vi "Facade.vi"(0 "Data In":T4, 2 "Display State In":T2, 3 "Container State":T3) -> (6 "Data Out":T4, 7 "Display State Out":T2, 8 "Action":T1)   [LabVIEW 2011, in "BlinkingButton.xctl"]
uses:
  <vilib>/_probes/SAPHIR/ViBox - Probes/BlinkingButton/BlinkingButton.xctl
  <vilib>/_probes/SAPHIR/ViBox - Probes/BlinkingButton/Data.ctl
  <vilib>/_xctls/Container State.ctl
  <vilib>/_probes/SAPHIR/ViBox - Probes/BlinkingButton/State.ctl
  <vilib>/_xctls/Action.ctl
  <vilib>/_xctls/XControlSupport.lvlib
panel:
  in  "FreezeDisplay":bool
  out "Blinker":bool
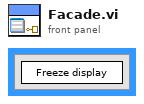
[diagram p1: front panel]
types:
  T1 = typedef "XControlSupport.lvlib/Action.ctl" = cluster{"Data Changed?":bool, "State Changed?":bool, "Action Name":string}
  T2 = typedef "BlinkingButton.xctl/State.ctl" = cluster{"Numeric":dbl}
  T3 = typedef "XControlSupport.lvlib/Container State.ctl" = cluster{"Indicator?":bool, "Run Mode?":bool, " Refnum":refnum<vi>}
  T4 = typedef "BlinkingButton.xctl/Data.ctl" = bool
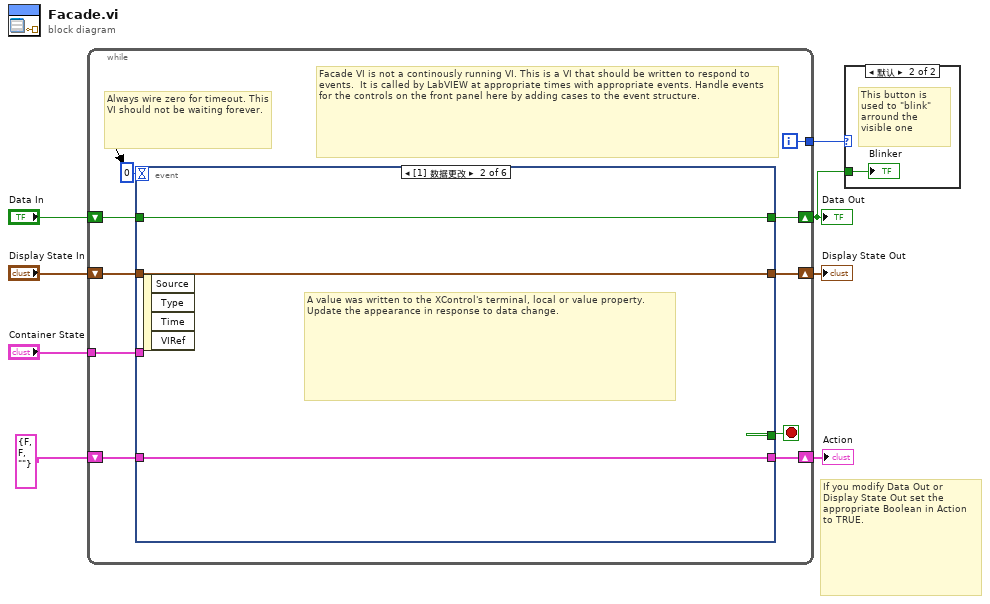
[diagram p0: block diagram]
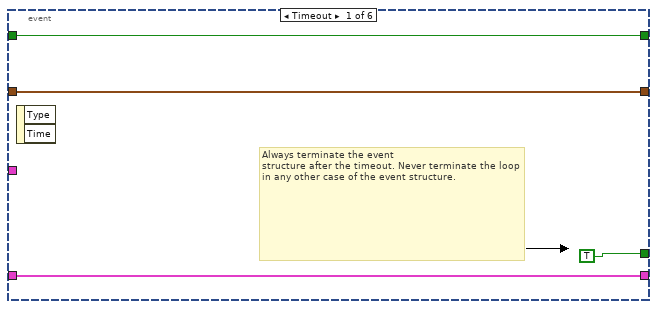
[diagram p3: hidden frame]
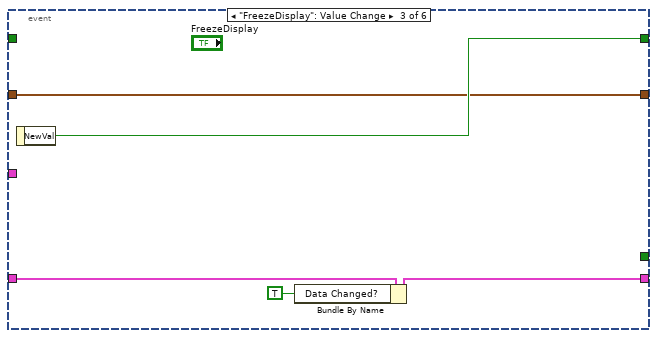
[diagram p4: hidden frame]
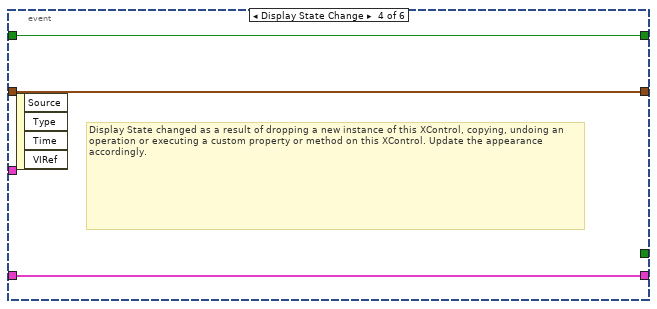
[diagram p5: hidden frame]
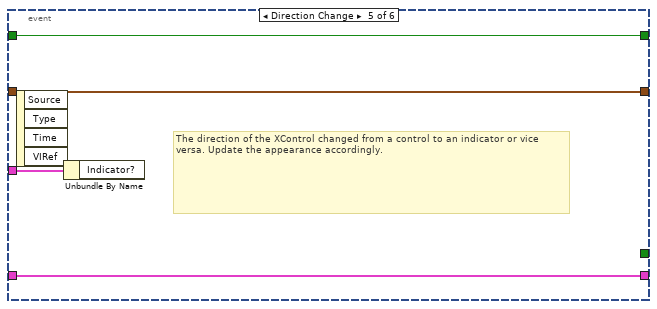
[diagram p6: hidden frame]
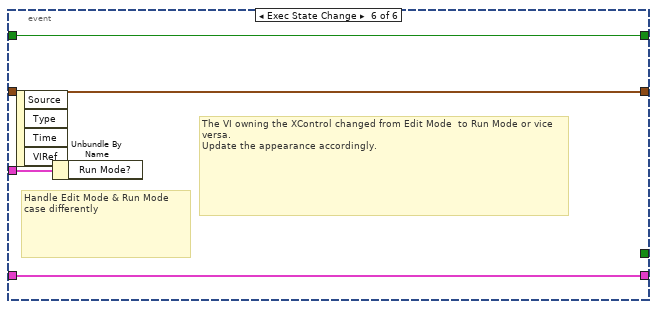
[diagram p7: hidden frame]
diagram:
  # "If you modify Data Out or\nDisplay State Out set the\nappropriate Boolean in Action\nto TRUE."
  n1 = while {
    shift-right: [w17] -> w6
    shift-left: "Display State In" -> [w18]
    tunnel: "Container State" -> [w14]
    shift-right: [w12] -> w1
    shift-left: "Data In" -> [w13]
    shift-right: [w10] -> w4
    shift-left: T1 {"Data Changed?"=FALSE, "State Changed?"=FALSE, "Action Name"=""} ("Action") -> [w11]
    tunnel: [w9] -> w2
    i -> [w9]
    stop <- w16 stop-if-true
    # "Facade VI is not a continously running VI. This is a VI that should be written to respond to events.  It is called by LabVIEW at appropriate times with appropriate events. Handle events for the controls on the front panel here by adding cases to the event structure."
    # "Always wire zero for timeout. This\nVI should not be waiting forever."
    n2 = event shown="[1] 数据更改" {
      selector: _ -> [_ _ _ _ _ _]
      dyn-events: _ -> [_ _ _ _ _ _]
      timeout: 0 -> [_ _ _ _ _ _]
      tunnel: w18 -> [w20 w24 w29 w33 w36 w40]
      tunnel: [w20 w24 w29 w33 w36 w40] -> w17
      tunnel: [TRUE _ _ _ _ _] -> w16
      tunnel: w14 -> [_ _ _ _ w37 w41]
      tunnel: w13 -> [w19 w25 _ w32 w35 w39]
      tunnel: [w19 w25 w30 w32 w35 w39] -> w12
      tunnel: [w21 w23 w28 w31 w34 w38] -> w10
      tunnel: w11 -> [w21 w23 w27 w31 w34 w38]
      event Timeout {
        # "Always terminate the event\nstructure after the timeout. Never terminate the loop in any other case of the event structure."
        n3 = event-data() -> ()  [unwired: 3 out]
      }
      event Data Change {
        # "A value was written to the XControl's terminal, local or value property.\nUpdate the appearance in response to data change."
        n4 = event-data() -> ()  [unwired: 5 out]
      }
      event "FreezeDisplay": Value Change {
        n5 = event-data() -> ("NewVal"=w30:bool)  [unwired: 1 out]
        n6 = Bundle By Name(cluster=w27, "Data Changed?"=TRUE) -> (w28:T1)
      }
      event Display State Change {
        # "Display State changed as a result of dropping a new instance of this XControl, copying, undoing an operation or executing a custom property or method on this XControl. Update the appearance accordingly."
        n7 = event-data() -> ()  [unwired: 5 out]
      }
      event Direction Change {
        # "The direction of the XControl changed from a control to an indicator or vice versa. Update the appearance accordingly."
        n8 = event-data() -> ()  [unwired: 5 out]
        n9 = Unbundle By Name(w37) -> ()  [unwired: 1 out]
      }
      event Exec State Change {
        # "The VI owning the XControl changed from Edit Mode  to Run Mode or vice versa.\nUpdate the appearance accordingly."
        # "Handle Edit Mode & Run Mode\ncase differently"
        n10 = event-data() -> ()  [unwired: 5 out]
        n11 = Unbundle By Name(w41) -> ()  [unwired: 1 out]
      }
    }
  }
  "Display State Out" <- w6
  "Data Out" <- w1
  "Action" <- w4
  n12 = case shown="默认" w2 {
    tunnel: w1 -> [_ w42]
    frame 0 {
    }
    frame Default {
      # "This button is used to \"blink\" arround the visible one"
      "Blinker" <- w42
    }
  }
